vi "Untitled 1 (SubVI).vi"   [LabVIEW 2020]
uses:
  HASO4_3/WaveKit/Classes/CorrectionDataManager/CorrectionDataManager.lvclass
  HASO4_3/WaveKit/Classes/Pupil/Pupil.lvclass
  HASO4_3/WaveKit/Controls/Point2Df.ctl
  HASO4_3/WaveKit/Controls/PupilDetectionMode.ctl
  HASO4_3/WaveKit/Controls/CircularAutoDetectionOptions.ctl
  HASO4_3/WaveKit/Controls/PupilDetectionOption.ctl
  HASO4_3/WaveKit/Controls/CircularPupilDetectionParams.ctl
  HASO4_3/WaveKit/Classes/ModalCoef/ModalCoef.lvclass
  HASO4_3/WaveKit/Controls/WavefrontModalReconstructionType.ctl
  HASO4_3/WaveKit/Classes/ComputePhaseSet/ComputePhaseSet.lvclass
  HASO4_3/WaveKit/Controls/WavefrontReconstructionMode.ctl
  HASO4_3/WaveKit/Classes/HasoSlopes/HasoSlopes.lvclass
  HASO4_3/WaveKit/Classes/WavefrontCorrector/WavefrontCorrector.lvclass
types:
  T1 = typedef "WavefrontReconstructionMode.ctl" = enum16{"None", "Modal_Legendre", "Modal_Zernike", "Zonal", "Modal_Zonal_Zernike", "Modal_Zonal_Legendre"}
  T2 = typedef "WavefrontModalReconstructionType.ctl" = enum16{"Legendre", "Zernike"}
  T3 = typedef "CircularPupilDetectionParams.ctl" = cluster{"PupilDetectionOption":T4, "AutoDetectionOption":T5, "PupilDetectionMode":T6, "CentralOccultationDetection":bool}
  T4 = typedef "PupilDetectionOption.ctl" = enum16{"Manual", "Automatic"}
  T5 = typedef "CircularAutoDetectionOptions.ctl" = enum16{"manual_radius_auto_center", "manual_center_auto_radius", "auto_radius_auto_center"}
  T6 = typedef "PupilDetectionMode.ctl" = enum16{"inscribed", "circumscribed"}
  T7 = typedef "Point2Df.ctl" = cluster{"X":sgl, "Y":sgl}
  T8 = typedef "CasaoManagerGeneralSpecifications.ctl" = cluster{"Wavefront corrector name":string, "Wavefront corrector serial number":string, "Nb actuators":i32, "HASO serial number":string, "Dimension_um":T9}
  T9 = typedef "General dimensions definition.ctl" = cluster{"Size":T10, "Step":T7}
  T10 = typedef "Point2D.ctl" = cluster{"X":u32, "Y":u32}
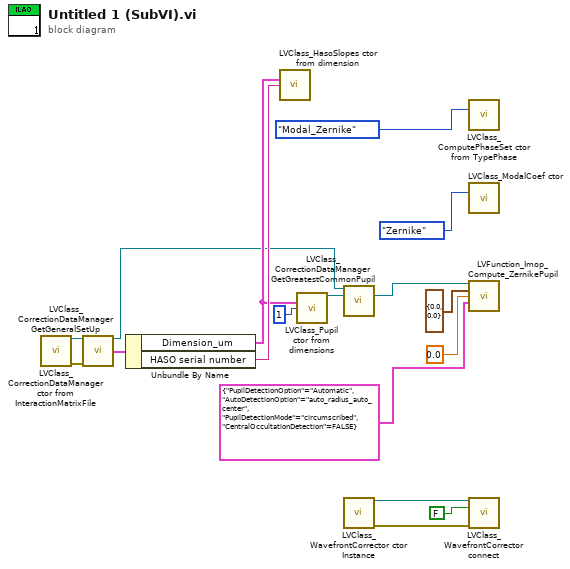
[diagram p0: block diagram]
diagram:
  n1 = call "LVClass_CorrectionDataManager ctor from InteractionMatrixFile.vi"() -> ("CorrectionDataManager (new)"=w1:refnum<class "CorrectionDataManager.lvclass">, "error out"=w2:errorcluster)  [unwired: 14 in]
  n2 = call "LVClass_CorrectionDataManager GetGeneralSetUp.vi"("CorrectionDataManager in"=w1, "error in (no error)"=w2) -> ("CorrectionDataManager out"=w4:refnum<class "CorrectionDataManager.lvclass">, "general"=w3:T8)  [unwired: 11 in, 1 out]
  n3 = Unbundle By Name(w3) -> ("Dimension_um"=w21:T9, "HASO serial number"=w22:string)
  n4 = call "LVClass_HasoSlopes ctor from dimension.vi"("Dimensions_um"=w21, "serial"=w22) -> ("HasoSlopes (const)"=w20:refnum<class "HasoSlopes.lvclass">, "HasoSlopes (new)"=w24:refnum<class "HasoSlopes.lvclass">)  [unwired: 11 in, 1 out]
  n5 = call "LVClass_Pupil ctor from dimensions.vi"("Dimensions_um"=w21, "value"=u8 1) -> ("Pupil (const)"=w5:refnum<class "Pupil.lvclass">, "Pupil (new)"=w7:refnum<class "Pupil.lvclass">)  [unwired: 11 in, 1 out]
  n6 = call "LVClass_CorrectionDataManager GetGreatestCommonPupil.vi"("CorrectionDataManager in"=w4, "Pupil in"=w7) -> ("CorrectionDataManager out"=w25:refnum<class "CorrectionDataManager.lvclass">, "Pupil out"=w11:refnum<class "Pupil.lvclass">)  [unwired: 11 in, 1 out]
  n7 = call "LVClass_WavefrontCorrector ctor Instance.vi"() -> ("WavefrontCorrector (const)"=w26:refnum<class "WavefrontCorrector.lvclass">, "WavefrontCorrector (new)"=w30:refnum<class "WavefrontCorrector.lvclass">, "PathToWavefrontCorrectorSetupFile"=w27:path, "error out"=w28:errorcluster)  [unwired: 12 in]
  n8 = call "LVClass_ComputePhaseSet ctor from TypePhase.vi"("TypePhase"=WavefrontReconstructionMode."Modal_Zernike") -> ("ComputePhaseSet (const)"=w19:refnum<class "ComputePhaseSet.lvclass">, "ComputePhaseSet (new)"=w23:refnum<class "ComputePhaseSet.lvclass">)  [unwired: 12 in, 1 out]
  n9 = call "LVClass_ModalCoef ctor.vi"("TypePhase"=WavefrontModalReconstructionType."Zernike") -> ("ModalCoef (const)"=w15:refnum<class "ModalCoef.lvclass">, "ModalCoef (new)"=w16:refnum<class "ModalCoef.lvclass">)  [unwired: 12 in, 1 out]
  n10 = call "LVFunction_Imop_Compute_ZernikePupil.vi"("Pupil.lvclass"=w11, "center in"=T7 {"X"=0.0, "Y"=0.0}, "radius in"=sgl 0.0, "CircularPupilDetectionParams"=T3 {"PupilDetectionOption"=enum."Automatic", "AutoDetectionOption"=enum."auto_radius_auto_center", "PupilDetectionMode"=enum."circumscribed", "CentralOccultationDetection"=FALSE}) -> ("Pupil.lvclass"=w17:refnum<class "Pupil.lvclass">, "center"=w12:T7, "radius"=w13:sgl)  [unwired: 8 in, 1 out]
  n11 = call "LVClass_WavefrontCorrector connect.vi"("WavefrontCorrector in"=w30, "set_init_state_from_config_file"=FALSE, "error in (no error)"=w28) -> ("WavefrontCorrector out"=w29:refnum<class "WavefrontCorrector.lvclass">)  [unwired: 11 in, 1 out]
